vi "Get Provided Interface and Service Class.vi"(8 "error in":errorcluster, 11 "session factory in":refnum<class "ISession Factory.lvclass">) -> (0 "error out":errorcluster, 1 "service class":string, 2 "provided interface":string, 3 "session factory out":refnum<class "ISession Factory.lvclass">)   [LabVIEW 2020, in "NI Session Management Instrument.lvlib" / "ISession Factory.lvclass"]
doc: "Returns the provided interface and service class that will be used to query the NI Discovery Service for the address and port of the instrument's gRPC server. If your instrument does not use a gRPC server then you do not have to override this VI."
uses:
  ISession Factory.lvclass
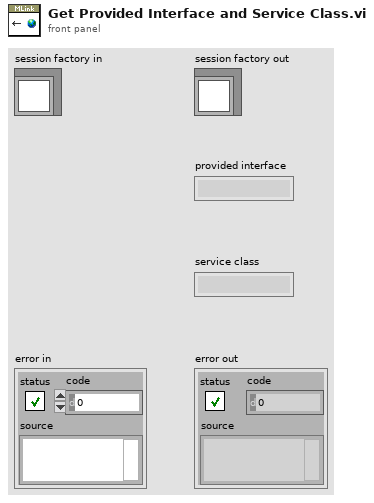
[diagram p1: front panel]
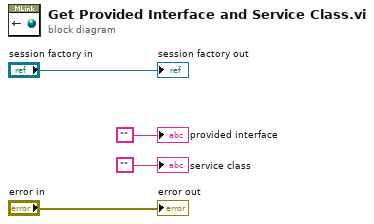
[diagram p0: block diagram]
diagram:
  "error out" <- "error in"
  "session factory out" <- "session factory in"
  "provided interface" <- "" ("grpc device interface")
  "service class" <- "" ("service class")
